vi "Raw FPGA Bus Controller Transmit.vi"() -> ()   [LabVIEW 2016]
uses:
  PPLs/FPGA Interface.lvlibp/FPGA Interface/FPGA Interface.lvclass
panel:
  in  "Stop":bool
  out "Data Transmitted":u16[](array[numeric]) format="%04x"
  in  "Word Count (1-32)":u16=32
  in  "Sub-Address (1-30)":u16=1
  in  "RT Address (0-30)":u16=1
  in  "Target Bus":enum16{"Bus B", "Bus A"}(ring)=enum."Bus A"
  in  "Transmit":bool
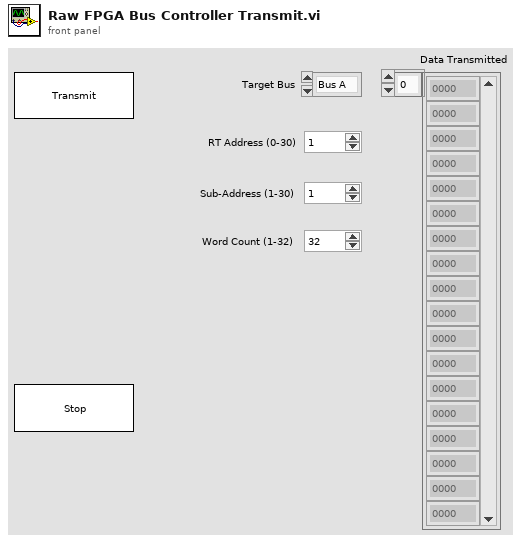
[diagram p1: front panel]
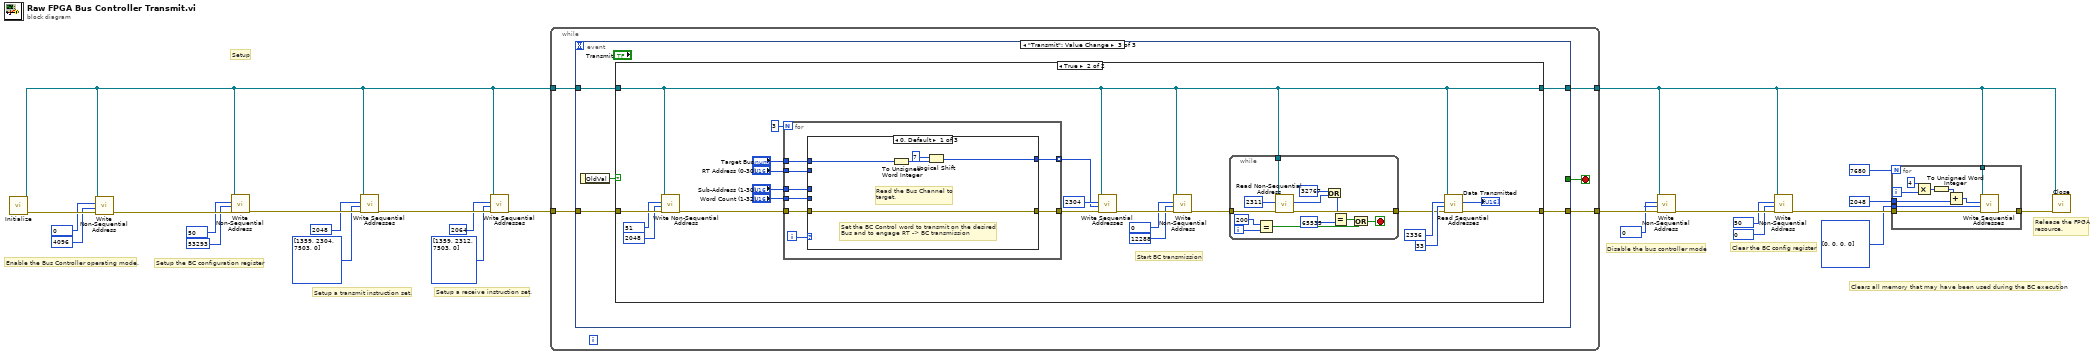
[diagram p0: block diagram]
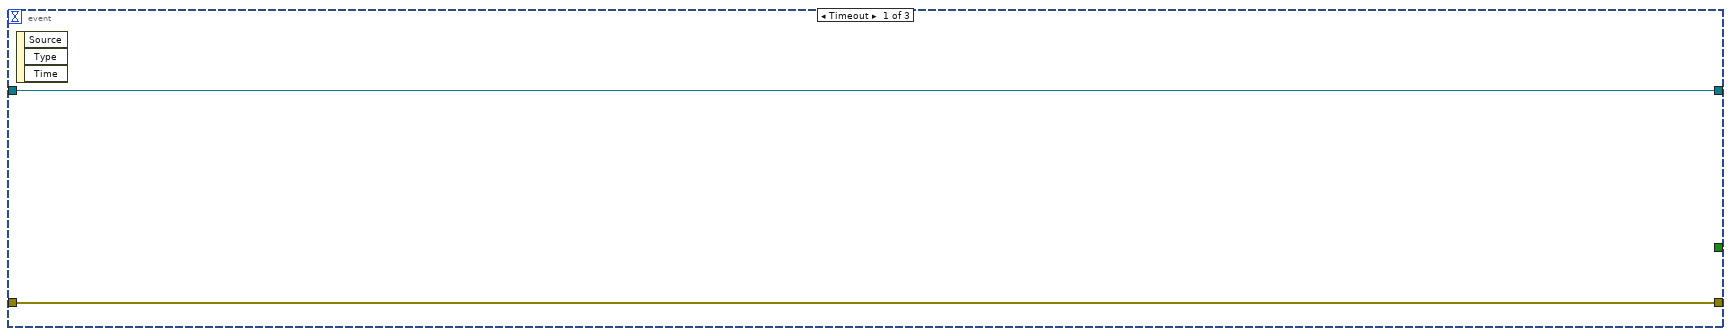
[diagram p2: hidden frame]
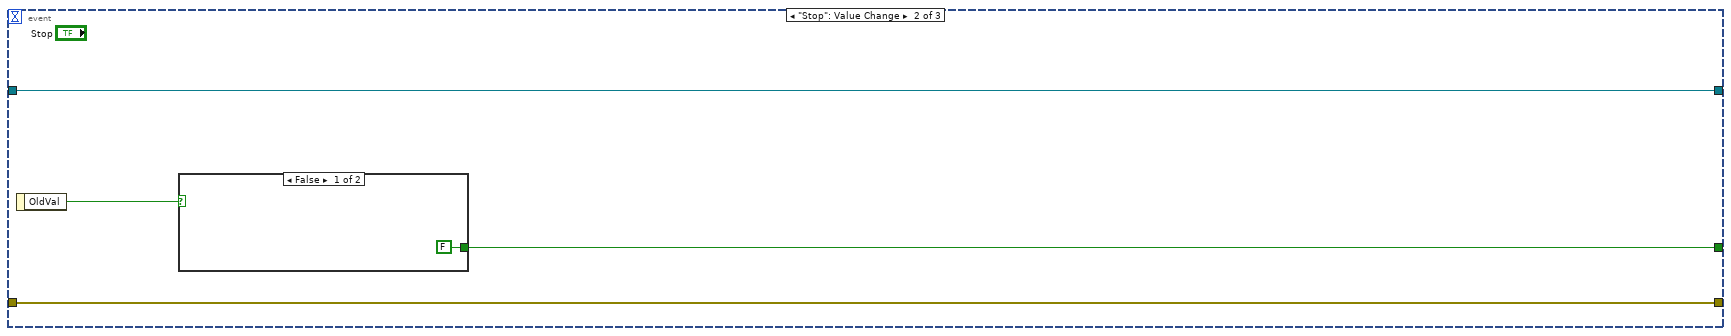
[diagram p3: hidden frame]
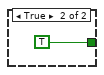
[diagram p4: hidden frame]
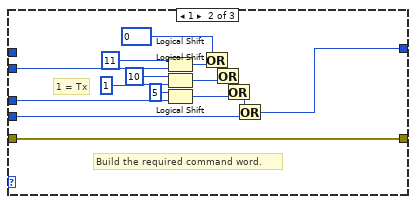
[diagram p6: hidden frame]
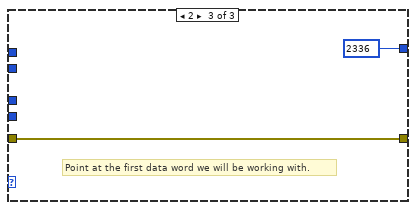
[diagram p7: hidden frame]
diagram:
  w10 = u16 0
  # "Release the FPGA\nresource."
  # "Clears all memory that may have been used during the BC execution"
  # "Clear the BC config register"
  # "Disable the bus controller mode"
  # "Setup"
  # "Setup a receive instruction set."
  # "Setup a transmit instruction set."
  # "Setup the BC configuration register"
  # "Enable the Bus Controller operating mode."
  n1 = call "Initialize.vi"() -> ("error out"=w25:errorcluster, "FPGA Interface out"=w12:refnum<class "FPGA Interface.lvclass">)  [unwired: 10 in]
  n2 = call-dynamic "Write Non-Sequential Address.vi"("error in (no error)"=w25, "Data"=u16 4096, "Address"=u16 0, "FPGA Interface in"=w12) -> ("error out"=w24:errorcluster)  [unwired: 7 in]
  n3 = call-dynamic "Write Non-Sequential Address.vi"("error in (no error)"=w24, "Data"=u16 53293, "Address"=u16 50, "FPGA Interface in"=w12) -> ("error out"=w23:errorcluster)  [unwired: 7 in]
  n4 = call-dynamic "Write Sequential Addresses.vi"("error in (no error)"=w23, "Data"=u16[] [1359, 2304, 7503, 0], "Starting Address"=u16 2048 ("Address"), "FPGA Interface in"=w12) -> ("error out"=w22:errorcluster)  [unwired: 7 in]
  n5 = call-dynamic "Write Sequential Addresses.vi"("error in (no error)"=w22, "Data"=u16[] [1359, 2312, 7503, 0], "Starting Address"=u16 2064 ("Address"), "FPGA Interface in"=w12) -> ("error out"=w13:errorcluster)  [unwired: 7 in]
  n6 = while {
    tunnel: w13 -> [w30]
    tunnel: w12 -> [w29]
    tunnel: [w28] -> w2
    tunnel: [w27] -> w11
    stop <- w26 stop-if-true
    n7 = event shown="[2] \"Transmit\": Value Change" {
      selector: _ -> [_ _ _]
      dyn-events: _ -> [_ _ _]
      timeout: _ -> [_ _ _]
      tunnel: w30 -> [w31 w34 w40]
      tunnel: w29 -> [w32 w36 w42]
      tunnel: [w32 w36 w43] -> w28
      tunnel: [w31 w34 w41] -> w27
      tunnel: [_ w33 _] -> w26
      event Timeout {
        n8 = event-data() -> ()  [unwired: 1 in, 3 out]
      }
      event "Stop": Value Change {
        n9 = event-data() -> ("OldVal"=w35:bool)  [unwired: 1 in]
        n10 = case shown="False" w35 {
          tunnel: [FALSE TRUE] -> w33
          frame False {
          }
          frame True {
          }
        }
      }
      event "Transmit": Value Change {
        n11 = event-data() -> ("OldVal"=w39:bool)  [unwired: 1 in]
        n12 = case shown="True" w39 {
          tunnel: [w45 w47] -> w43
          tunnel: w42 -> [w45 w47]
          tunnel: [w44 w49] -> w41
          tunnel: w40 -> [w44 w67]
          frame False {
          }
          frame True {
            # "Start BC transmission"
            n13 = call-dynamic "Write Non-Sequential Address.vi"("error in (no error)"=w67, "Data"=u16 2048, "Address"=u16 51, "FPGA Interface in"=w47) -> ("error out"=w64:errorcluster)  [unwired: 7 in]
            n14 = for {
              N: 3 -> [_]
              tunnel: w64 -> [w87]
              tunnel: [w88] -> w58
              tunnel: "Target Bus" -> [w85]
              tunnel: "RT Address (0-30)" -> [w84]
              tunnel: "Sub-Address (1-30)" -> [w83]
              tunnel: "Word Count (1-32)" -> [w82]
              tunnel: [w81] -> w56 mode=indexing
              i -> [w86]
              n15 = case shown="0, Default" w86 {
                tunnel: [w93 w109 w111] -> w88
                tunnel: w87 -> [w93 w109 w111]
                tunnel: w85 -> [w91 _ _]
                tunnel: w84 -> [_ w98 _]
                tunnel: w83 -> [_ w97 _]
                tunnel: w82 -> [_ w96 _]
                tunnel: [w89 w94 u16 2336 ("Address")] -> w81
                frame 0, Default {
                  # "Read the Bus Channel to\ntarget."
                  # "Set the BC Control word to transmit on the desired\nBus and to engage RT -> BC transmission"
                  n16 = To Unsigned Word Integer(number=w91) -> (unsigned 16bit integer=w90:u16)
                  n17 = Logical Shift(y=i16 7, x=w90) -> (x << y=w89:u16)
                }
                frame 1 {
                  # "1 = Tx"
                  # "Build the required command word."
                  n18 = Logical Shift(y=i16 11, x=w98) -> (x << y=w105:u16)
                  n19 = Logical Shift(y=i16 10, x=u16 1 ("Tx/Rx")) -> (x << y=w104:u16)
                  n20 = Logical Shift(y=i16 5, x=w97) -> (x << y=w101:u16)
                  n21 = Or(x=u16 0 ("Address"), y=w105) -> (x .or. y?=w103:u16)
                  n22 = Or(x=w103, y=w104) -> (x .or. y?=w102:u16)
                  n23 = Or(x=w102, y=w101) -> (x .or. y?=w100:u16)
                  n24 = Or(x=w100, y=w96) -> (x .or. y?=w94:u16)
                }
                frame 2 {
                  # "Point at the first data word we will be working with."
                }
              }
            }
            n25 = call-dynamic "Write Sequential Addresses.vi"("error in (no error)"=w58, "Data"=w56, "Starting Address"=u16 2304 ("Address"), "FPGA Interface in"=w47) -> ("error out"=w55:errorcluster)  [unwired: 7 in]
            n26 = call-dynamic "Write Non-Sequential Address.vi"("error in (no error)"=w55, "Data"=u16 12288, "Address"=u16 0, "FPGA Interface in"=w47) -> ("error out"=w52:errorcluster)  [unwired: 7 in]
            n27 = while {
              tunnel: w52 -> [w79]
              tunnel: [w78] -> w48
              tunnel: w47 -> [w80]
              i -> [w74]
              stop <- w71 stop-if-true
              n28 = Equal?(x=200, y=w74) -> (x = y?=w75:bool)
              n29 = call-dynamic "Read Non-Sequential Address.vi"("error in (no error)"=w79, "Address"=u16 2311, "FPGA Interface in"=w80) -> ("error out"=w78:errorcluster, "Data"=w69:u16)  [unwired: 7 in]
              n30 = Or(x=u16 32767 ("Address"), y=w69) -> (x .or. y?=w68:u16)
              n31 = Equal?(x=w68, y=u16 65535 ("Address")) -> (x = y?=w77:bool)
              n32 = Or(x=w77, y=w75) -> (x .or. y?=w71:bool)
            }
            n33 = call-dynamic "Read Sequential Addresses.vi"("error in (no error)"=w48, "Addresses to Read"=33, "Starting Address"=u16 2336 ("Address"), "FPGA Interface in"=w47) -> ("error out"=w49:errorcluster, "Data"=→"Data Transmitted":u16[])  [unwired: 6 in]
          }
        }
      }
    }
  }
  n34 = call-dynamic "Write Non-Sequential Address.vi"("error in (no error)"=w11, "Data"=w10, "Address"=w10, "FPGA Interface in"=w2) -> ("error out"=w9:errorcluster)  [unwired: 7 in]
  n35 = call-dynamic "Write Non-Sequential Address.vi"("error in (no error)"=w9, "Data"=u16 0, "Address"=u16 50, "FPGA Interface in"=w2) -> ("error out"=w6:errorcluster)  [unwired: 7 in]
  n36 = for {
    N: 7680 -> [_]
    tunnel: w2 -> [w121]
    tunnel: w6 -> [w120]
    tunnel: u16[] [0, 0, 0, 0] ("Data") -> [w119]
    tunnel: u16 2048 -> [w114]
    tunnel: [w112] -> w1
    i -> [w115]
    n37 = Multiply(x=4, y=w115) -> (x*y=w117:i32)
    n38 = To Unsigned Word Integer(number=w117) -> (unsigned 16bit integer=w116:u16)
    n39 = Add(x=w116, y=w114) -> (x+y=w113:u16)
    n40 = call-dynamic "Write Sequential Addresses.vi"("error in (no error)"=w120, "Data"=w119, "Starting Address"=w113, "FPGA Interface in"=w121) -> ("error out"=w112:errorcluster)  [unwired: 7 in]
  }
  n41 = call "Close.vi"("error in (no error)"=w1, "FPGA Interface in"=w2) -> ()  [unwired: 9 in, 1 out]
